vi "Read Single Measurement.vi"   [LabVIEW 2019, in "Agilent 681x Series.lvlib"]
doc: "Initiates and reads the selected single measurement.\n\n<B>Note:</B>\n\nThis VI changes the <B>Trigger Source</B> to <B>Bus</B> and uses a software trigger after the instrument is initiated. If you want to control the triggering and other features, please use the low level VIs."
uses:
  <instrlib>/Agilent 681x Series/Agilent 681x Series.lvlib
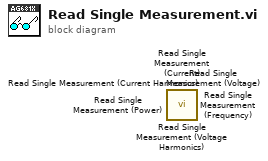
[diagram p0: block diagram]
diagram:
  n1 = call <instrlib>:"Read Single Measurement (Voltage Harmonics).vi"() -> ()  [unwired: 11 in, 5 out]
  n2 = call <instrlib>:"Read Single Measurement (Voltage).vi"() -> ()  [unwired: 11 in, 5 out]
  n3 = call <instrlib>:"Read Single Measurement (Power).vi"() -> ()  [unwired: 8 in, 8 out]
  n4 = call <instrlib>:"Read Single Measurement (Frequency).vi"() -> ()  [unwired: 13 in, 3 out]
  n5 = call <instrlib>:"Read Single Measurement (Current Harmonics).vi"() -> ()  [unwired: 10 in, 6 out]
  n6 = call <instrlib>:"Read Single Measurement (Current).vi"() -> ()  [unwired: 10 in, 6 out]
